vi "Send Stop Command To Robot.vi"() -> ()   [LabVIEW 2016]
uses:
  Communication Global variables.vi
  <vilib>/addons/_JKI.lib/REST Client/classes/REST Client/REST Client.lvclass
panel:
  out "error out":errorcluster
  in  "error in (no error)":errorcluster
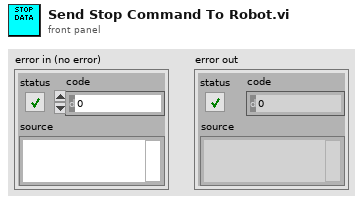
[diagram p1: front panel]
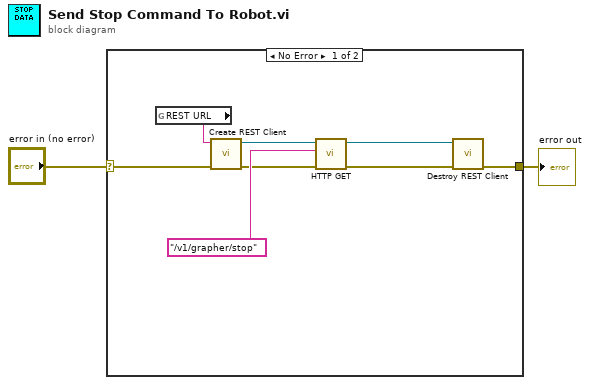
[diagram p0: block diagram]
diagram:
  n1 = case shown="No Error" "error in (no error)" {
    selector: "error in (no error)" -> [w10 w11]
    tunnel: [w3 w11] -> w1
    frame No Error {
      n2 = global read "Communication Global variables.vi" "REST URL"() -> (w5:string)
      n3 = call <vilib>:"Create REST Client.vi"("error in (no error)"=w10, "Base URL"=w5) -> ("error out"=w7:errorcluster, "REST Client out"=w9:refnum<class "REST Client.lvclass">)  [unwired: 8 in]
      n4 = call-dynamic "HTTP GET.vi"("error in (no error)"=w7, "Path"="/v1/grapher/stop", "REST Client in"=w9) -> ("error out"=w4:errorcluster, "REST Client out"=w6:refnum<class "REST Client.lvclass">)  [unwired: 3 in, 4 out]
      n5 = call-dynamic "Destroy REST Client.vi"("error in (no error)"=w4, "REST Client in"=w6) -> ("error out"=w3:errorcluster)  [unwired: 9 in]
    }
    frame Error {
    }
  }
  "error out" <- w1
